vi "Main.vi"(11 "Module Admin":refnum<class "Delacor_lib_QMH_Module Admin.lvclass">) -> ()   [LabVIEW 2021, in "Sequence Engine.lvlib"]
doc: "This template is based off of the Queued Message Handler design pattern and the Queued Message Handler project template that ships with LabVIEW.\n\nThe main difference is that the queue is private to this module and communication between modules is performed via Broadcast and Request events.\n\nRequest events are wrapped in public API methods and are handled in the Event Handling Loop (EHL) of this VI. Any module can register for Broadcast events sent by this module. The EHL generates messages based on user interface actions.\n\nThe Message Handling Loop (MHL) processes messages generated by the EHL, or by other messages. The messages are string values, so new messages can be added easily to the Message Cases case structure in the MHL. Each message cluster can also provide an optional value for Message Data, which is a variant that can be converted to whatever message-specific data is required.\n_____\nBased on DQMH Dev Tools: Project Template 7.1.1.1528."
uses:
  Sequence Engine.lvlib
  <vilib>/Delacor/Delacor QMH/Libraries/Module Admin_class/Delacor_lib_QMH_Module Admin.lvclass
  Module Data--cluster.ctl
  Classes/Test Step/Test Step.lvclass
  Classes/Test Result/Test Result.lvclass
  Classes/Sequence Engine/Sequence Engine.lvclass
  Classes/Results Manager/Results Manager.lvclass
  Classes/UUT/UUT.lvclass
  <vilib>/Delacor/Delacor QMH/Libraries/Message Queue_class/Delacor_lib_QMH_Message Queue.lvclass/Delacor_lib_QMH_Message Queue.ctl
  Stop Argument--cluster.ctl
  <vilib>/Delacor/Delacor QMH/Libraries/Module Admin_class/Delacor_lib_QMH_Module Admin.lvclass/Delacor_lib_QMH_Module Admin.ctl
  REQ Run Sequence Argument--cluster.ctl
  Init Test Context Argument--cluster.ctl
  Sequence Context.ctl
  <vilib>/Utility/miscctls.llb/LVPointTypeDef.ctl
  Classes/Sequence Engine/Sequence Engine.lvclass/Sequence Engine.ctl
  Classes/UUT/UUT.lvclass/UUT.ctl
  Classes/Test Result/Result Data.ctl
  Classes/Test Result/Test Status.ctl
  Classes/Test Result/Test Result.lvclass/Test Result.ctl
  <vilib>/Delacor/Delacor QMH/Libraries/Message Queue_class/Delacor_lib_QMH_Enqueue Message (Single).vi
  <vilib>/Delacor/Delacor QMH/Libraries/Module Admin_class/Delacor_lib_QMH_Get External Launch.vi
  <vilib>/Delacor/Delacor QMH/Libraries/Message Queue_class/Delacor_lib_QMH_Message Queue.lvclass
  PPLs/Recipe.lvlibp/Classes/Recipe/Recipe.lvclass
panel:
  out "error out":errorcluster
  out "Status":string
  in  "Simulate MHL Error":bool
  in  "Simulate EHL Error":bool
  # "Other processes communicate with this Module via its Public API (wrappers for its Request Events).\n\nThis Module communicates with other processes via its Broadcast Events.\nAny process that wants to receive these messages can register for this module's Broadcast events."
  # "This template is for the DQMH framework. See the block diagram for more information on how to use this template."
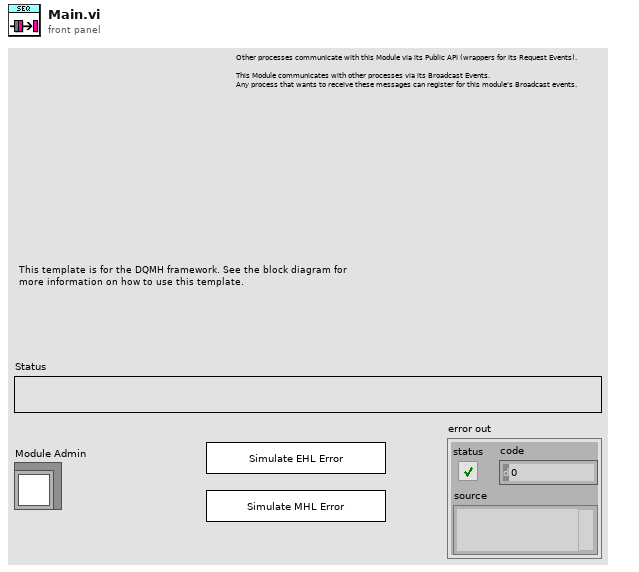
[diagram p1: front panel]
types:
  T1 = typedef "Sequence Engine.lvlib/Request Events--cluster.ctl" = cluster{"Stop Module":refnum<user-event>, "Show Panel":refnum<user-event>, "Hide Panel":refnum<user-event>, "Get Module Execution Status":refnum<user-event>, "Show Diagram":refnum<user-event>, "REQ Run Sequence":refnum<user-event>, "Request to stop testing":refnum<user-event>, "Init Test Context":refnum<user-event>}
  T2 = typedef "Sequence Engine.lvlib/Module Data--cluster.ctl" = cluster{"Steps Array":refnum<class "Test Step.lvclass">[], "Status":string, "Current Index":i32, "Current Step":refnum<class "Test Step.lvclass">, "Retried Count":u8, "Test Result":refnum<class "Test Result.lvclass">, "Sequence Engine":refnum<class "Sequence Engine.lvclass">, "Is Fail":bool, "Results Manager":refnum<class "Results Manager.lvclass">, "UUT.lvclass":refnum<class "UUT.lvclass">, "Run.Start JSON":string, "Test Aborted":bool}
  T3 = enum32{"invalid lock state", "Not Locked", "Locked (No Password)", "Password-protected"}
  T4 = typedef "Sequence Engine.lvlib/Stop Argument--cluster.ctl" = cluster{"Origin":string, "Exit via Stop Module Req?":bool, "Wait for Module to stop?":bool}
  T5 = typedef "Sequence Engine.lvlib/REQ Run Sequence Argument--cluster.ctl" = cluster{"Run.Start JSON":string}
  T6 = typedef "Sequence Engine.lvlib/Init Test Context Argument--cluster.ctl" = cluster{"Sequence Context":T7}
  T7 = typedef "Sequence Engine.lvlib/Sequence Engine.lvclass/Sequence Context.ctl" = cluster{"Execution Mode":enum16{"Production", "MSA1", "Trial"}, "Username":string, "Is Simulation":bool, "Hardware Map":string}
  T8 = typedef "LVPointTypeDef.ctl" = cluster{"Horizontal":i16, "Vertical":i16}
  T9 = enum32{"Invalid", "Standard", "Closed", "Hidden", "Minimized", "Maximized"}
  T10 = typedef "Sequence Engine.lvlib/Test Result.lvclass/Result Data.ctl" = cluster{"Test ID":u32, "Test Name":string, "Sub Test Name":string, "Test Status":T11, "Start Time":timestamp, "End Time":timestamp, "Duration (s)":dbl, "Expected Values":string, "Measured Values":string, "Remarks":string}
  T11 = typedef "Sequence Engine.lvlib/Test Result.lvclass/Test Status.ctl" = enum16{"Pass", "Fail", "Aborted", "Skipped"}
  T12 = typedef "Sequence Engine.lvlib/Test Factory.lvclass/Test Config.ctl" = cluster{"Test ID":string, "Test Name":string, "Test Group":string, "Enabled?":bool, "Timeout (s)":u16, "Retry Count":u16, "Recipe Parameters":string, "Sequence Config":string}
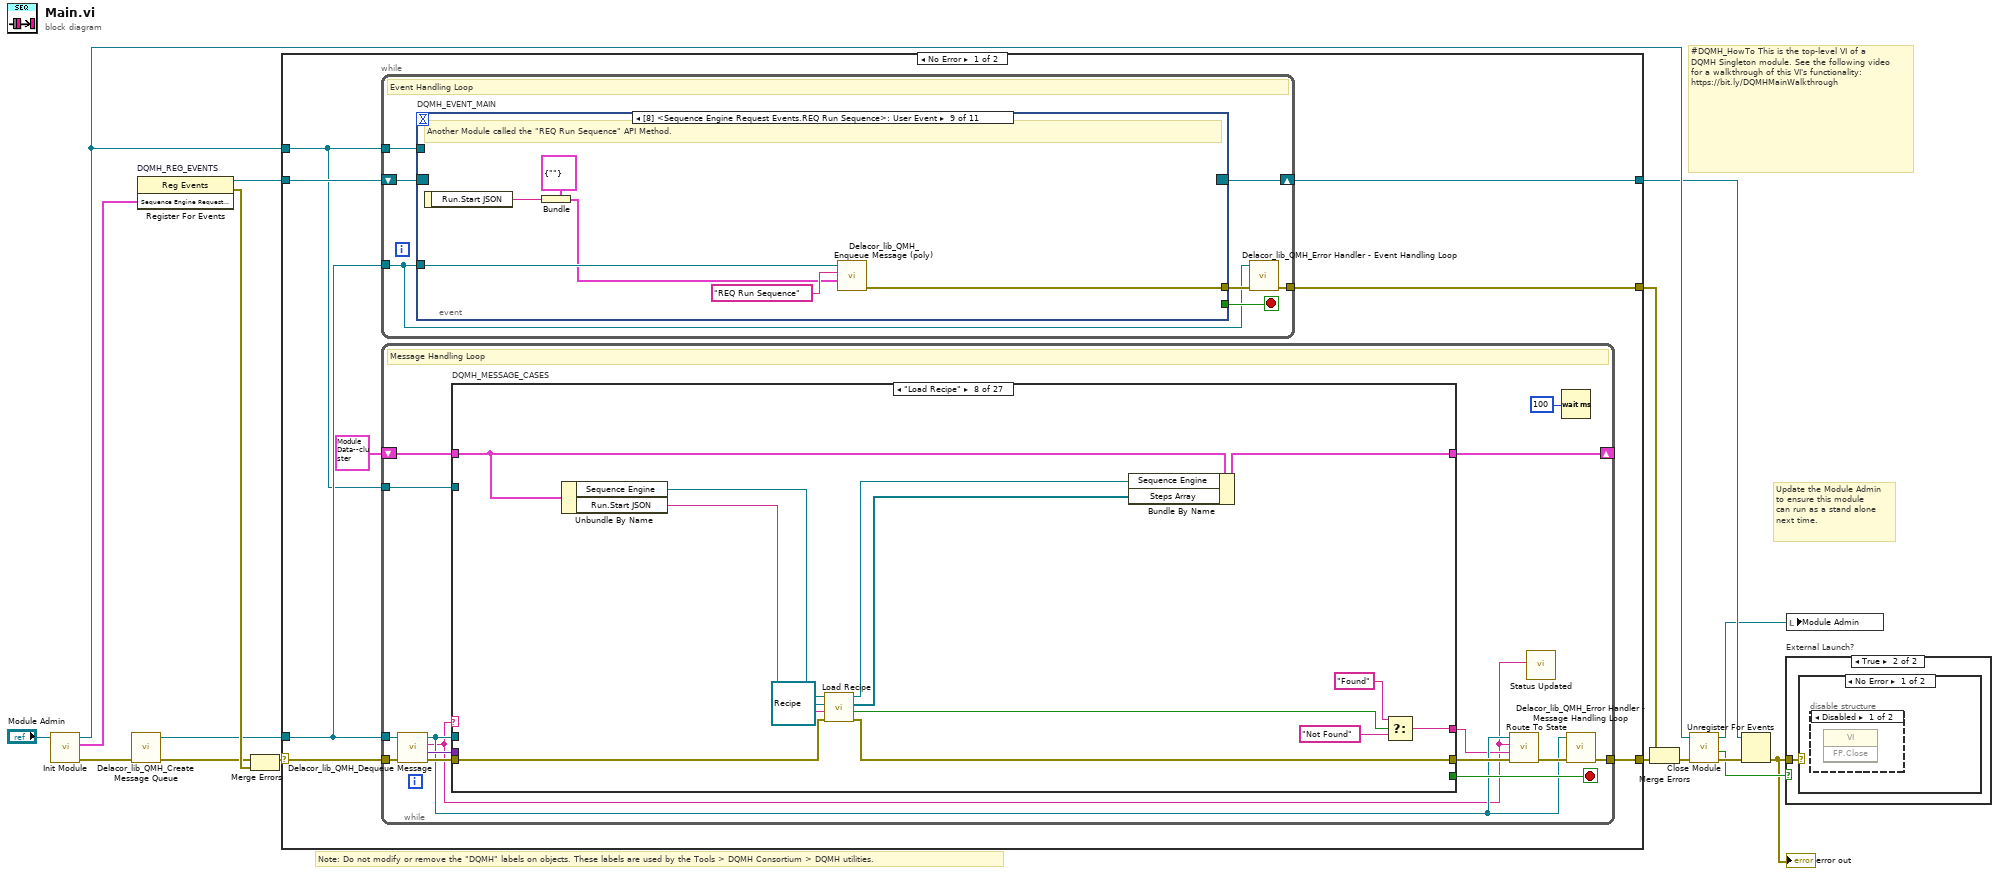
[diagram p0: block diagram]
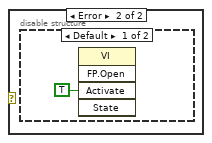
[diagram p4: hidden frame]
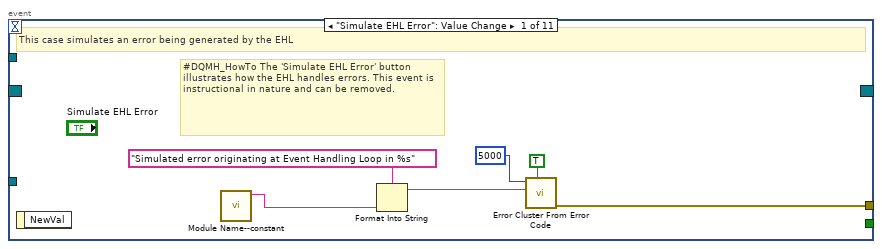
[diagram p6: hidden frame]
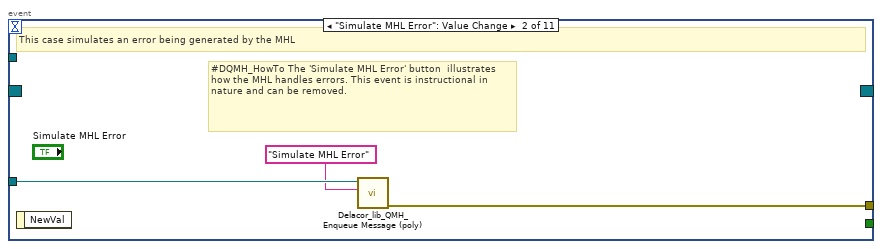
[diagram p7: hidden frame]
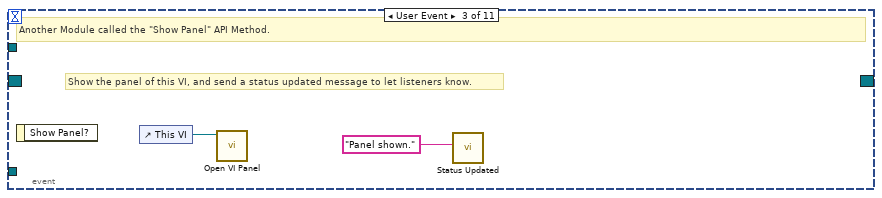
[diagram p8: hidden frame]
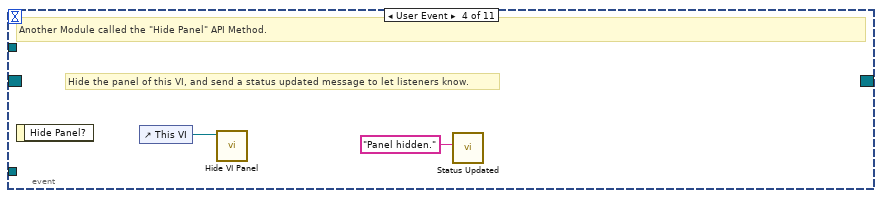
[diagram p9: hidden frame]
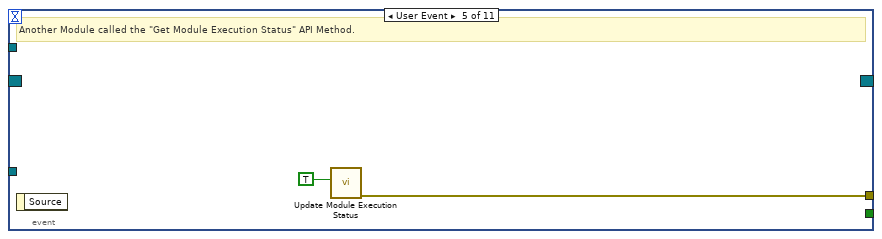
[diagram p10: hidden frame]
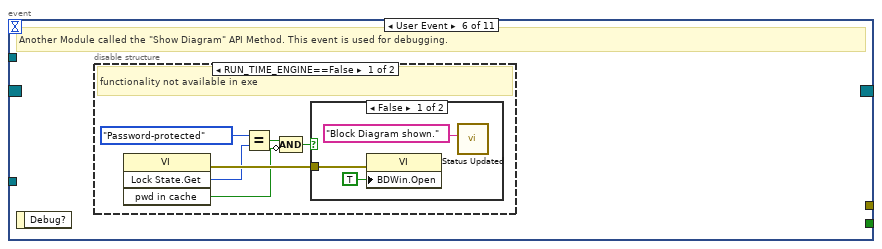
[diagram p11: hidden frame]
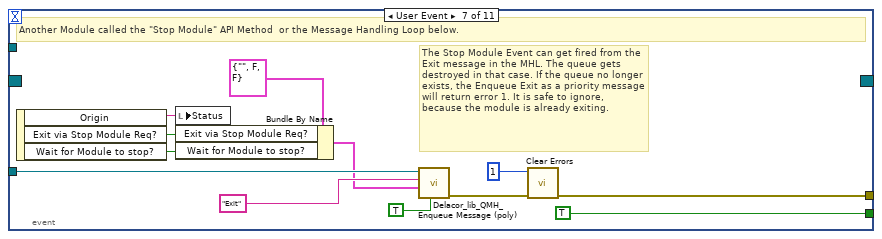
[diagram p14: hidden frame]
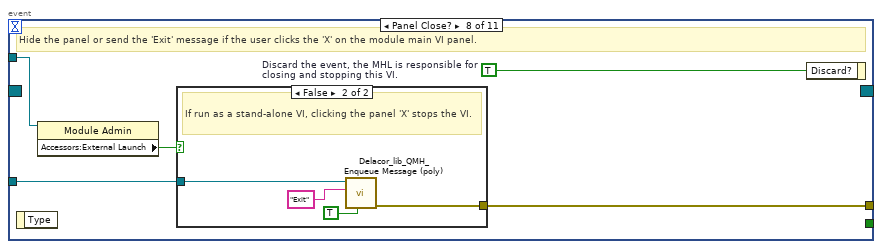
[diagram p15: hidden frame]
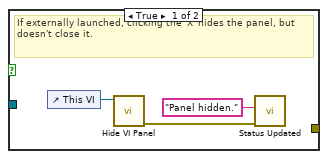
[diagram p16: hidden frame]
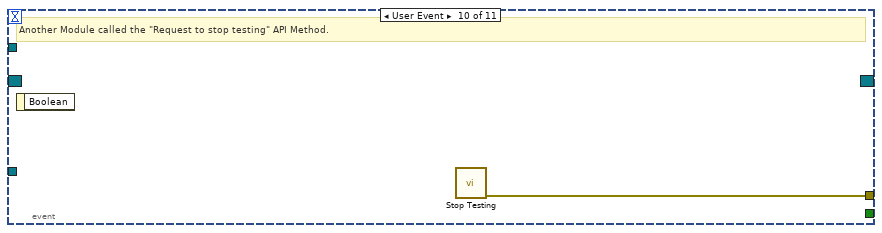
[diagram p17: hidden frame]
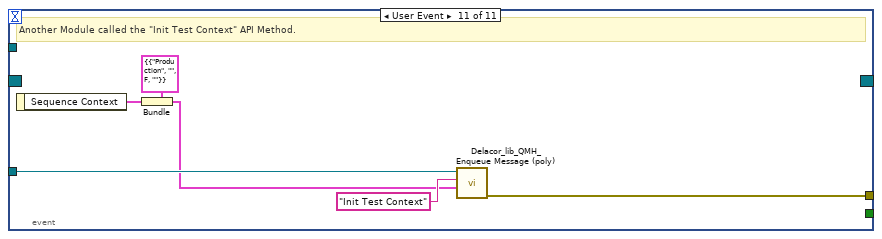
[diagram p18: hidden frame]
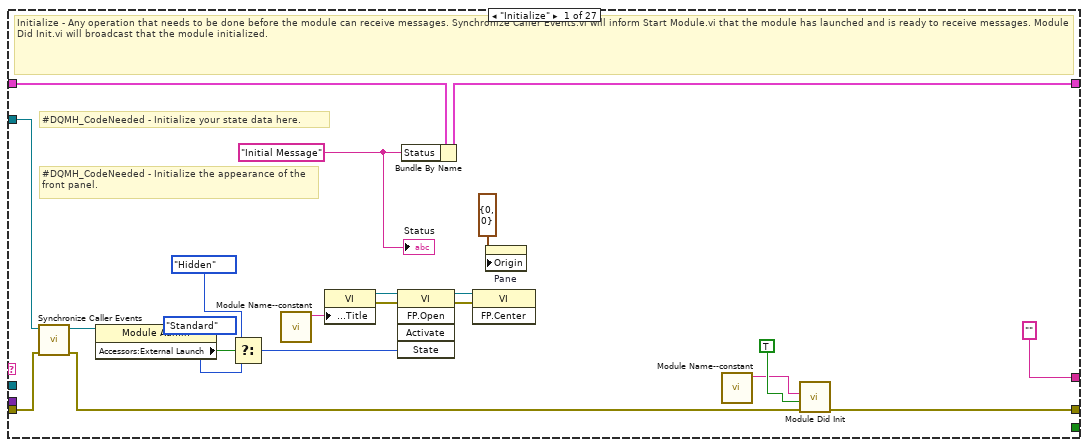
[diagram p19: hidden frame]
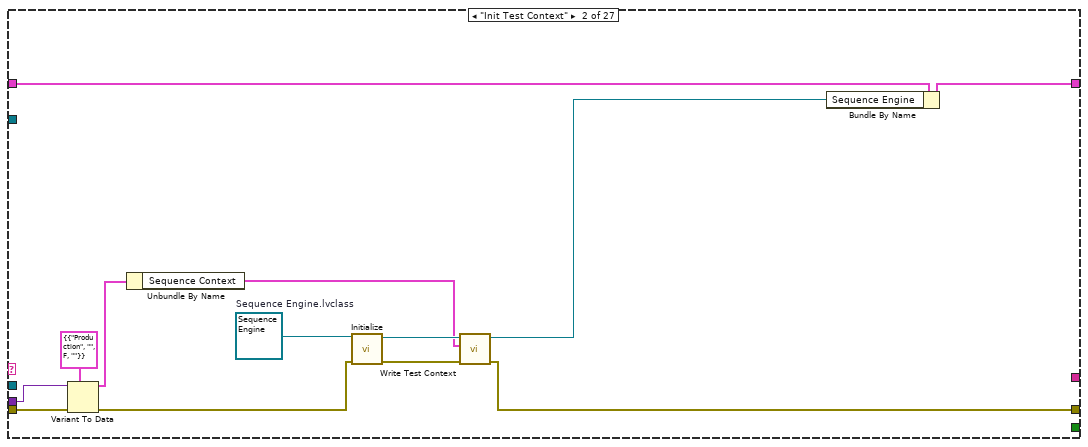
[diagram p20: hidden frame]
diagram:
  # "#DQMH_HowTo This is the top-level VI of a DQMH Singleton module. See the following video for a walkthrough of this VI's functionality: https://bit.ly/DQMHMainWalkthrough"
  # "Note: Do not modify or remove the \"DQMH\" labels on objects. These labels are used by the Tools > DQMH Consortium > DQMH utilities."
  # "Update the Module Admin to ensure this module can run as a stand alone next time."
  n1 = call "Init Module.vi"("Singleton Module Admin in"="Module Admin") -> ("error out"=w3:errorcluster, "Sequence Engine Request Events"=w8:T1, "Singleton Module Admin out"=w11:refnum<class "Delacor_lib_QMH_Module Admin.lvclass">)  [unwired: 8 in]
  n2 = call <vilib>:"Delacor_lib_QMH_Create Message Queue.vi"("error in"=w3) -> ("error out"=w2:errorcluster, "Message Queue"=w4:refnum<class "Delacor_lib_QMH_Message Queue.lvclass">)  [unwired: 9 in]
  n3 = register-events "DQMH_REG_EVENTS"(w8) -> (reference out=w9:refnum<event-registration>, error out=w12:errorcluster)  [unwired: 2 in]
  n4 = Merge Errors(w2, w12) -> (w13:errorcluster)
  n5 = case shown="No Error" w13 {
    selector: w13 -> [w23 w374]
    tunnel: [w25 w373] -> w17
    tunnel: [w22 w372] -> w10
    tunnel: w9 -> [w21 w372]
    tunnel: w4 -> [w20 w367]
    tunnel: [w24 _] -> w15
    tunnel: w11 -> [w19 w368]
    frame No Error {
      n6 = while {
        tunnel: w20 -> [w26]
        shift-right: [w29] -> w22
        shift-left: w21 -> [w30]
        tunnel: [w31] -> w24
        tunnel: w19 -> [w27]
        stop <- w28 stop-if-true
        # "Event Handling Loop"
        n7 = event "DQMH_EVENT_MAIN" shown="[8] <Sequence Engine Request Events.REQ Run Sequence>: User Event" {
          selector: w30 -> [_ _ _ _ _ _ _ _ _ _ _]
          dyn-events: [_ _ _ _ _ _ _ _ _ _ _] -> w29
          timeout: _ -> [_ _ _ _ _ _ _ _ _ _ _]
          tunnel: [_ _ _ _ _ _ TRUE ("Discard?") _ _ _ _] -> w28
          tunnel: w26 -> [_ w40 _ _ _ _ w64 w71 w86 _ w93]
          tunnel: [w38 w41 _ _ w47 _ w67 w73 w81 w87 w88] -> w32
          tunnel: w27 -> [_ _ _ _ _ _ _ w70 _ _ _]
          event "Simulate EHL Error": Value Change {
            # "#DQMH_HowTo The 'Simulate EHL Error' button  illustrates how the EHL handles errors. This event is instructional in nature and can be removed."
            # "This case simulates an error being generated by the EHL"
            n8 = event-data() -> ()  [unwired: 1 in, 1 out]
            n9 = call "Module Name--constant.vi"() -> ("Module Name"=w35:string)  [unwired: 11 in]
            n10 = Format Into String(format string="Simulated error originating at Event Handling Loop in %s", w35) -> (resulting string=w36:string)  [unwired: 2 in, 1 out]
            n11 = call <vilib>:"Error Cluster From Error Code.vi"("show call chain? (False)"=TRUE, "error message (\"\")"=w36, "error code (0)"=5000) -> ("error out"=w38:errorcluster)  [unwired: 6 in]
          }
          event "Simulate MHL Error": Value Change {
            # "#DQMH_HowTo The 'Simulate MHL Error' button  illustrates how the MHL handles errors. This event is instructional in nature and can be removed."
            # "This case simulates an error being generated by the MHL"
            n12 = event-data() -> ()  [unwired: 1 in, 1 out]
            n13 = call-poly <vilib>:"Delacor_lib_QMH_Enqueue Message (poly).vi"("Message"="Simulate MHL Error", "Message Queue in"=w40) -> ("error out"=w41:errorcluster)  [unwired: 8 in, 1 out]
          }
          event User Event {
            # "Show the panel of this VI, and send a status updated message to let listeners know."
            # "Another Module called the \"Show Panel\" API Method."
            n14 = event-data() -> ()  [unwired: 1 in, 1 out]
            n15 = control-ref of="This VI"() -> (w43:refnum<vi>)
            n16 = call "Open VI Panel.vi"("VI"=w43) -> ()  [unwired: 10 in, 1 out]
            n17 = call "Status Updated.vi"("Status"="Panel shown." ("format string")) -> ()  [unwired: 10 in, 1 out]
          }
          event User Event {
            # "Hide the panel of this VI, and send a status updated message to let listeners know."
            # "Another Module called the \"Hide Panel\" API Method."
            n18 = event-data() -> ()  [unwired: 1 in, 1 out]
            n19 = control-ref of="This VI"() -> (w45:refnum<vi>)
            n20 = call "Hide VI Panel.vi"("VI"=w45) -> ()  [unwired: 10 in, 1 out]
            n21 = call "Status Updated.vi"("Status"="Panel hidden." ("format string")) -> ()  [unwired: 10 in, 1 out]
          }
          event User Event {
            # "Another Module called the \"Get Module Execution Status\" API Method."
            n22 = event-data() -> ()  [unwired: 1 in, 1 out]
            n23 = call "Update Module Execution Status.vi"("Running?"=TRUE) -> ("error out"=w47:errorcluster)  [unwired: 10 in]
          }
          event User Event {
            # "Another Module called the \"Show Diagram\" API Method. This event is used for debugging."
            n24 = event-data() -> ()  [unwired: 1 in, 1 out]
            n25 = disable-structure shown="RUN_TIME_ENGINE==False" {
              frame condition #0 (active) {
                # "functionality not available in exe"
                n26 = invoke on="Invoke Node" class="VI" method="Lock State.Get"() -> (error out=w53:errorcluster, "Get Lock State"=w52:T3, "pwd in cache"=w49:bool)  [unwired: 4 in, 1 out]
                n27 = Equal?(x=T3."Password-protected", y=w52) -> (x = y?=w50:bool)
                n28 = Compound Arithmetic op=AND(w50, invert w49) -> (w48:bool)
                n29 = case shown="False" w48 {
                  tunnel: w53 -> [w56 _]
                  frame False {
                    n30 = property on="Property Node" class="VI"(error in=w56, "BDWin.Open"=TRUE ("Block Diagram Window:Open")) -> ()  [unwired: 1 in, 2 out]
                    n31 = call "Status Updated.vi"("Status"="Block Diagram shown." ("format string")) -> ()  [unwired: 10 in, 1 out]
                  }
                  frame True {
                    # "Password-protected VI, and the password is not in the cache. Do not show the diagram."
                  }
                }
              }
              frame condition #1 {
              }
            }
          }
          event User Event {
            # "The Stop Module Event can get fired from the Exit message in the MHL. The queue gets destroyed in that case. If the queue no longer exists, the Enqueue Exit as a priority message will return error 1. It is safe to ignore, because the module is already exiting."
            # "Another Module called the \"Stop Module\" API Method  or the Message Handling Loop below."
            n32 = event-data() -> ("Origin"=w63:string, "Exit via Stop Module Req?"=w59:bool, "Wait for Module to stop?"=w58:bool)  [unwired: 1 in]
            n33 = local write "Status"(w63) -> ()
            n34 = Bundle By Name(cluster=T4 {"Origin"="", "Exit via Stop Module Req?"=FALSE, "Wait for Module to stop?"=FALSE} ("Stop Argument"), "Exit via Stop Module Req?"=w59, "Wait for Module to stop?"=w58) -> (w57:T4)
            n35 = call-poly <vilib>:"Delacor_lib_QMH_Enqueue Message (poly).vi"("Priority Message? (F)"=TRUE, "Message Data"=w57, "Message"="Exit", "Message Queue in"=w64) -> ("error out"=w68:errorcluster)  [unwired: 6 in, 1 out]
            n36 = call <vilib>:"Clear Errors.vi"("error in (no error)"=w68, "specific error code to clear (0: all)"=1) -> ("error out"=w67:errorcluster)  [unwired: 4 in, 1 out]
          }
          event Panel Close? {
            w72 = TRUE  # Discard the event, the MHL is responsible for closing and stopping this VI.
            # "Hide the panel or send the 'Exit' message if the user clicks the 'X' on the module main VI panel."
            n37 = event-data() -> ()  [unwired: 1 in, 1 out]
            n38 = property on="Property Node" class="Module Admin"(reference=w70) -> ("Accessors:External Launch"=w69:bool)  [unwired: 1 in, 2 out]
            n39 = case shown="False" w69 {
              tunnel: w71 -> [_ w79]
              tunnel: [_ w80] -> w73
              frame True {
                # "If externally launched, clicking the 'X' hides the panel, but doesn't close it."
                n40 = control-ref of="This VI"() -> (w76:refnum<vi>)
                n41 = call "Hide VI Panel.vi"("VI"=w76) -> ("error out"=w74:errorcluster)  [unwired: 10 in]
                n42 = call "Status Updated.vi"("error in"=w74, "Status"="Panel hidden." ("format string")) -> ()  [unwired: 9 in, 1 out]
              }
              frame False {
                # "If run as a stand-alone VI, clicking the panel 'X' stops the VI."
                n43 = call-poly <vilib>:"Delacor_lib_QMH_Enqueue Message (poly).vi"("Priority Message? (F)"=TRUE, "Message"="Exit", "Message Queue in"=w79) -> ("error out"=w80:errorcluster)  [unwired: 7 in, 1 out]
              }
            }
            n44 = event-data ("Event Filter Node")("Discard?"=w72) -> ()  [unwired: 1 in, 1 out]
          }
          event User Event {
            # "Another Module called the \"REQ Run Sequence\" API Method."
            n45 = event-data() -> ("Run.Start JSON"=w82:string)  [unwired: 1 in]
            n46 = Bundle(cluster=T5 {"Run.Start JSON"=""} ("REQ Run Sequence Argument"), "Run.Start JSON"=w82) -> (w83:T5)
            n47 = call-poly <vilib>:"Delacor_lib_QMH_Enqueue Message (poly).vi"("Message Data"=w83, "Message"="REQ Run Sequence", "Message Queue in"=w86) -> ("error out"=w81:errorcluster)  [unwired: 7 in, 1 out]
          }
          event User Event {
            # "Another Module called the \"Request to stop testing\" API Method."
            n48 = event-data() -> ()  [unwired: 1 in, 1 out]
            n49 = call "Stop Testing.vi"() -> ("error out"=w87:errorcluster)  [unwired: 11 in]
          }
          event User Event {
            # "Another Module called the \"Init Test Context\" API Method."
            n50 = event-data() -> ("Sequence Context"=w89:T7)  [unwired: 1 in]
            n51 = Bundle(cluster=T6 {"Sequence Context"={"Execution Mode"=enum."Production", "Username"="", "Is Simulation"=FALSE, "Hardware Map"=""}} ("Init Test Context Argument"), "Sequence Context"=w89) -> (w90:T6)
            n52 = call-poly <vilib>:"Delacor_lib_QMH_Enqueue Message (poly).vi"("Message Data"=w90, "Message"="Init Test Context", "Message Queue in"=w93) -> ("error out"=w88:errorcluster)  [unwired: 7 in, 1 out]
          }
        }
        n53 = call-dynamic "Delacor_lib_QMH_Error Handler - Event Handling Loop.vi"("error in"=w32, "Message Queue in"=w26) -> ("dup error in"=w31:errorcluster)  [unwired: 8 in, 1 out]
      }
      n54 = while {
        tunnel: w20 -> [w100]
        shift-right: [w105] -> _
        shift-left: T2 {"Steps Array"=[], "Status"="", "Current Index"=0, "Current Step"=refnum, "Retried Count"=0, "Test Result"=refnum, "Sequence Engine"=refnum, "Is Fail"=FALSE, "Results Manager"=refnum, "UUT.lvclass"=refnum, "Run.Start JSON"="", "Test Aborted"=FALSE} ("Module Data") -> [w106]
        tunnel: w23 -> [w108]
        tunnel: [w101] -> w25
        tunnel: w19 -> [w102]
        stop <- w104 stop-if-true
        # "Message Handling Loop"
        n55 = call-dynamic "Delacor_lib_QMH_Dequeue Message.vi"("error in"=w108, "Message Queue in"=w100) -> ("error out"=w107:errorcluster, "Message Data"=w103:variant, "Message"=w95:string, "Message Queue out"=w97:refnum<class "Delacor_lib_QMH_Message Queue.lvclass">)  [unwired: 6 in]
        n56 = case "DQMH_MESSAGE_CASES" shown="\"Load Recipe\"" w95 {
          selector: w95 -> [_ _ _ _ _ _ _ _ _ _ _ _ _ _ _ _ _ _ _ _ _ _ _ _ _ _ w362]
          tunnel: w97 -> [_ _ _ _ _ _ _ _ _ _ _ _ _ _ _ _ _ _ _ _ _ _ _ _ w327 w351 _]
          tunnel: w107 -> [w127 w142 w144 w153 w157 w159 w162 w172 w182 w191 w203 w213 w227 w230 w248 w267 w275 w279 w295 w303 w309 w312 w314 w323 w334 w356 w365]
          tunnel: [w126 w130 w144 w152 w157 w159 w162 w171 w177 w191 w203 w213 w226 w229 w246 w262 w275 w278 w288 w302 w309 w311 w314 w322 w330 w341 w366] -> w99
          tunnel: w106 -> [w117 w141 w143 w155 w156 w158 w163 w176 w184 w190 w202 w212 w225 w242 w251 w272 w274 w282 w294 w307 w308 w310 w313 w320 w329 w342 w363]
          tunnel: [w116 w134 w143 w151 w156 w158 w161 w174 w181 w190 w201 w210 w223 w236 w247 w273 w274 w282 w289 w306 w308 w310 w313 w320 w329 w342 w363] -> w105
          tunnel: [_ _ _ _ _ _ _ _ _ _ _ _ _ _ _ _ _ _ _ _ _ _ _ _ _ w350 _] -> w104
          tunnel: w103 -> [_ w140 _ w147 _ _ _ _ _ _ _ _ _ _ _ _ _ _ _ _ _ _ _ _ w328 w349 _]
          tunnel: w102 -> [w118 _ _ _ _ _ _ _ _ _ _ _ _ _ _ _ _ _ _ _ _ _ _ _ w326 w344 _]
          tunnel: ["" ("Outcome") _ _ _ _ _ _ w168 _ _ w193 _ w218 w237 _ w255 _ w281 _ _ _ _ _ _ _ _ _] -> w96
          frame "Initialize" {
            w112 = "Initial Message" ("Initial Message")
            # "#DQMH_CodeNeeded - Initialize the appearance of the front panel."
            # "#DQMH_CodeNeeded - Initialize your state data here."
            # "Initialize - Any operation that needs to be done before the module can receive messages. Synchronize Caller Events.vi will inform Start Module.vi that the module has launched and is ready to receive messages. Module Did Init.vi will broadcast that the module initialized."
            n57 = call "Synchronize Caller Events.vi"("error in"=w127, "Singleton Module Admin in"=w118) -> ("error out"=w110:errorcluster, "Singleton Module Admin out"=w113:refnum<class "Delacor_lib_QMH_Module Admin.lvclass">)  [unwired: 8 in]
            n58 = property on="Property Node" class="Module Admin"(reference=w113) -> ("Accessors:External Launch"=w122:bool)  [unwired: 1 in, 2 out]
            n59 = Select(t=T9."Hidden" ("State"), s=w122, f=T9."Standard" ("State")) -> (s? t:f=w119:T9)
            n60 = call "Module Name--constant.vi"() -> ("Module Name"=w125:string)  [unwired: 11 in]
            n61 = property on="Property Node" class="VI"("Front Panel.Title"=w125) -> (reference out=w124:refnum<vi>, error out=w129:errorcluster)  [unwired: 2 in]
            n62 = invoke on="Invoke Node" class="VI" method="FP.Open"(reference=w124, error in=w129, "State"=w119) -> (reference out=w123:refnum<vi>, error out=w128:errorcluster)  [unwired: 2 in, 3 out]
            n63 = Bundle By Name(cluster=w117, "Status"=w112) -> (w116:T2)
            n64 = invoke on="Invoke Node" class="VI" method="FP.Center"(reference=w123, error in=w128) -> ()  [unwired: 1 in, 3 out]
            n65 = property on="Pane" class="Pane"("Origin"=T8 {"Horizontal"=0, "Vertical"=0}) -> ()  [unwired: 2 in, 2 out]
            n66 = call "Module Name--constant.vi"() -> ("Module Name"=w114:string)  [unwired: 11 in]
            n67 = call "Module Did Init.vi"("error in"=w110, "Initialized?"=TRUE, "Origin"=w114) -> ("error out"=w126:errorcluster)  [unwired: 8 in]
            "Status" <- w112
          }
          frame "Init Test Context" {
            w135 = refnum<class "Sequence Engine.lvclass"> refnum  # Sequence Engine.lvclass
            n68 = Variant To Data(error in=w142, type=T6 {"Sequence Context"={"Execution Mode"=enum."Production", "Username"="", "Is Simulation"=FALSE, "Hardware Map"=""}} ("Init Test Context Argument"), Variant=w140) -> (data=w138:T6, error out=w132:errorcluster)
            n69 = Unbundle By Name(w138) -> ("Sequence Context"=w131:T7)
            n70 = call "Initialize.vi"("error in (no error)"=w132, "Sequence Engine in"=w135) -> ("error out"=w137:errorcluster, "Sequence Engine out"=w136:refnum<class "Sequence Engine.lvclass">)  [unwired: 8 in]
            n71 = call "Write Test Context.vi"("error in (no error)"=w137, "Test Context"=w131, "Sequence Engine in"=w136) -> ("error out"=w130:errorcluster, "Sequence Engine out"=w133:refnum<class "Sequence Engine.lvclass">)  [unwired: 7 in]
            n72 = Bundle By Name(cluster=w141, "Sequence Engine"=w133) -> (w134:T2)
          }
          frame "---Module Specific---" {
            # "Separator -- The following cases handle messages specific to this Module."
          }
          frame "REQ Run Sequence" {
            n73 = Variant To Data(error in=w153, type=T5 {"Run.Start JSON"=""} ("REQ Run Sequence Argument"), Variant=w147) -> (data=w146:T5, error out=w149:errorcluster)
            n74 = Unbundle By Name(w146) -> ("Run.Start JSON"=w145:string)
            n75 = Unbundle By Name(w155) -> ("Sequence Engine"=w154:refnum<class "Sequence Engine.lvclass">)
            n76 = call "Run.vi"("error in (no error)"=w149, "Sequence Engine in"=w154) -> ("error out"=w152:errorcluster, "Sequence Engine out"=w150:refnum<class "Sequence Engine.lvclass">)  [unwired: 8 in]
            n77 = Bundle By Name(cluster=w155, "Sequence Engine"=w150, "Run.Start JSON"=w145) -> (w151:T2)
          }
          frame "---Sequence Specific---" {
            # "Separator -- The following cases handle messages specific to this Test Sequence"
          }
          frame "--- UUT Loop starts ----" {
          }
          frame "Pre Sequence Run" {
            n78 = Bundle By Name(cluster=w163, "Current Index"=0) -> (w161:T2)
          }
          frame "Load Recipe" {
            n79 = Unbundle By Name(w176) -> ("Sequence Engine"=w175:refnum<class "Sequence Engine.lvclass">, "Run.Start JSON"=w169:string)
            n80 = call "Load Recipe.vi"("error in (no error)"=w172, "Run.Start JSON"=w169, "Recipe.lvclass"=refnum<class "Recipe.lvclass"> refnum, "Sequence Engine in"=w175) -> ("error out"=w171:errorcluster, "Found?"=w165:bool, "Steps Array"=w173:refnum<class "Test Step.lvclass">[], "Sequence Engine out"=w170:refnum<class "Sequence Engine.lvclass">)  [unwired: 4 in]
            n81 = Bundle By Name(cluster=w176, "Sequence Engine"=w170, "Steps Array"=w173) -> (w174:T2)
            n82 = Select(t="Found", s=w165, f="Not Found") -> (s? t:f=w168:string)
          }
          frame "Insert Report Header" {
            n83 = Unbundle By Name(w184) -> ("Sequence Engine"=w183:refnum<class "Sequence Engine.lvclass">, "UUT.lvclass"=w179:refnum<class "UUT.lvclass">)
            n84 = disable-structure shown="Disabled" {
              disable-tunnel: w183 -> [w189 _]
              disable-tunnel: w182 -> [w188 _]
              disable-tunnel: [w187 _] -> w180
              disable-tunnel: w179 -> [w186 _]
              disable-tunnel: [w185 _] -> w178
              frame Disabled {
                n85 = call "Create Report Header.vi"("error in (no error)"=w188, "UUT.lvclass"=w186, "Sequence Engine in"=w189) -> ("error out"=w185:errorcluster, "Sequence Engine out"=w187:refnum<class "Sequence Engine.lvclass">)  [unwired: 6 in, 1 out]
              }
              frame Enabled {
              }
            }
            n86 = call "Testing Started.vi"("error in"=w178) -> ("error out"=w177:errorcluster)  [unwired: 10 in]
            n87 = Bundle By Name(cluster=w184, "Sequence Engine"=w180) -> (w181:T2)
          }
          frame "--- Test Loop starts ----" {
          }
          frame "Sequence Iterator" {
            n88 = Unbundle By Name(w202) -> ("Steps Array"=w199:refnum<class "Test Step.lvclass">[], "Current Index"=w198:i32)
            n89 = Index Array(array=w199, index=w198) -> (element=w200:refnum<class "Test Step.lvclass">)
            n90 = Array Size(array=w199) -> (size(s)=w197:i32)
            n91 = Less?(x=w198, y=w197) -> (x < y?=w196:bool)
            n92 = Select(t="Pre Test", s=w196, f="Completed") -> (s? t:f=w193:string)
            n93 = Bundle By Name(cluster=w202, "Retried Count"=u8 0, "Current Step"=w200) -> (w201:T2)
          }
          frame "Pre Test Run" {
            n94 = Unbundle By Name(w212) -> ("Current Step"=w211:refnum<class "Test Step.lvclass">)
            n95 = Get Date/Time In Seconds() -> (seconds since 1Jan1904=w205:timestamp)
            n96 = Bundle By Name(cluster=T10 {"Test ID"=0, "Test Name"="", "Sub Test Name"="", "Test Status"=enum."Pass", "Start Time"=timestamp(0 s since 1904-01-01), "End Time"=timestamp(0 s since 1904-01-01), "Duration (s)"=0.0, "Expected Values"="", "Measured Values"="", "Remarks"=""} ("Result Data"), "Start Time"=w205) -> (w206:T10)
            n97 = call "Write Result Data.vi"("Result Data"=w206, "Test Result in"=refnum<class "Test Result.lvclass"> refnum ("Test Result.lvclass")) -> ("Test Result out"=w204:refnum<class "Test Result.lvclass">)  [unwired: 8 in, 1 out]
            n98 = call-dynamic "Init Test Result Data.vi"("Result.lvclass"=w204, "Test Step in"=w211) -> ("Test Step out"=w209:refnum<class "Test Step.lvclass">)  [unwired: 8 in, 1 out]
            n99 = Bundle By Name(cluster=w212, "Current Step"=w209) -> (w210:T2)
          }
          frame "Execute Test" {
            n100 = Unbundle By Name(w225) -> ("Current Step"=w224:refnum<class "Test Step.lvclass">)
            n101 = call-dynamic "Execute.vi"("error in (no error)"=w227, "Test Step in"=w224) -> ("error out"=w226:errorcluster, "Test Result"=w221:refnum<class "Test Result.lvclass">, "Test Step out"=w222:refnum<class "Test Step.lvclass">)  [unwired: 7 in]
            n102 = call "Read Result Data.vi"("Test Result in"=w221) -> ("Result Data"=w219:T10)  [unwired: 8 in, 2 out]
            n103 = Unbundle By Name(w219) -> ("Test Status"=w215:T11)
            n104 = call "New Test Result.vi"("Result Data"=w219) -> ()  [unwired: 10 in, 1 out]
            n105 = Equal?(x=Test_Status."Aborted", y=w215) -> (x = y?=w214:bool)
            n106 = Equal?(x=Test_Status."Fail", y=w215) -> (x = y?=w217:bool)
            n107 = Bundle By Name(cluster=w225, "Current Step"=w222, "Test Result"=w221, "Test Aborted"=w214, "Is Fail"=w217) -> (w223:T2)
            n108 = Format Into String(w215) -> (resulting string=w218:string)  [unwired: 3 in, 1 out]
          }
          frame "Test Fail" {
            n109 = Unbundle By Name(w242) -> ("Retried Count"=w233:u8, "Current Step"=w241:refnum<class "Test Step.lvclass">)
            n110 = call-dynamic "Read Step Config.vi"("error in (no error)"=w230, "Test Step in"=w241) -> ("Step Config"=w240:T12)  [unwired: 7 in, 2 out]
            n111 = Unbundle By Name(w240) -> ("Retry Count"=w228:u16)
            n112 = To Unsigned Word Integer(number=w233) -> (unsigned 16bit integer=w231:u16)
            n113 = call "Retried Count.vi"("error in"=w230, "Retried Count"=w228) -> ("error out"=w229:errorcluster)  [unwired: 9 in]
            n114 = Greater?(x=w228, y=w231) -> (0:w235:bool)
            n115 = Increment(x=w233) -> (x+1=w234:u8)
            n116 = Select(t="Retry", s=w235, f="Don't Retry") -> (s? t:f=w237:string)
            n117 = Select(t=w234, s=w235, f=w233) -> (s? t:f=w232:u8)
            n118 = Bundle By Name(cluster=w242, "Retried Count"=w232) -> (w236:T2)
          }
          frame "Save Test Result" {
            n119 = Unbundle By Name(w251) -> ("Sequence Engine"=w245:refnum<class "Sequence Engine.lvclass">, "Test Aborted"=w243:bool, "Current Step"=w250:refnum<class "Test Step.lvclass">)
            n120 = disable-structure shown="Disabled" {
              disable-tunnel: w250 -> [w254 _]
              disable-tunnel: [w253 _] -> w249
              disable-tunnel: w248 -> [w252 _]
              frame Disabled {
                n121 = call-dynamic "Save Test Result.vi"("error in (no error)"=w252, "Test Step in"=w254) -> ("error out"=w253:errorcluster)  [unwired: 8 in, 1 out]
              }
              frame Enabled {
              }
            }
            n122 = call "Write Is Aborted.vi"("error in (no error)"=w249, "Is Aborted"=w243, "Sequence Engine in"=w245) -> ("error out"=w246:errorcluster, "Sequence Engine out"=w244:refnum<class "Sequence Engine.lvclass">)  [unwired: 7 in]
            n123 = Bundle By Name(cluster=w251, "Sequence Engine"=w244) -> (w247:T2)
          }
          frame "Post Test Run" {
            n124 = Unbundle By Name(w272) -> ("Current Index"=w271:i32, "Results Manager"=w269:refnum<class "Results Manager.lvclass">, "Test Result"=w268:refnum<class "Test Result.lvclass">, "Sequence Engine"=w266:refnum<class "Sequence Engine.lvclass">, "Test Aborted"=w257:bool, "Is Fail"=w261:bool)
            n125 = Increment(x=w271) -> (x+1=w270:i32)
            n126 = call-dynamic "Add Result.vi"("error in (no error)"=w267, "Test Result.lvclass"=w268, "Results Manager in"=w269) -> ("error out"=w263:errorcluster, "Results Manager out"=w265:refnum<class "Results Manager.lvclass">)  [unwired: 7 in]
            n127 = call "Write Results Manager.vi"("error in (no error)"=w263, "Results Manager.lvclass"=w265, "Sequence Engine in"=w266) -> ("error out"=w262:errorcluster, "Sequence Engine out"=w264:refnum<class "Sequence Engine.lvclass">)  [unwired: 7 in]
            n128 = Bundle By Name(cluster=w272, "Current Index"=w270, "Results Manager"=w265, "Sequence Engine"=w264) -> (w273:T2)
            n129 = Select(t="Test Fail", s=w261, f="Not Fail") -> (s? t:f=w258:string)
            n130 = Select(t="Test Aborted", s=w257, f=w258) -> (s? t:f=w255:string)
          }
          frame "--- Test Loop stops ----" {
          }
          frame "Check Execution Mode" {
            n131 = Unbundle By Name(w282) -> ("Sequence Engine"=w280:refnum<class "Sequence Engine.lvclass">)
            n132 = call "Read Test Context.vi"("error in (no error)"=w279, "Sequence Engine in"=w280) -> ("error out"=w278:errorcluster, "Test Context"=w277:T7)  [unwired: 7 in, 1 out]
            n133 = Unbundle By Name(w277) -> ("Execution Mode"=w276:enum16{"Production", "MSA1", "Trial"})
            n134 = case shown="\"Production\", Default" w276 {
              tunnel: ["Production"] -> w281
              frame "Production", Default {
              }
            }
          }
          frame "Save Final Result" {
            n135 = Unbundle By Name(w294) -> ("Results Manager"=w290:refnum<class "Results Manager.lvclass">, "Sequence Engine"=w292:refnum<class "Sequence Engine.lvclass">, "UUT.lvclass"=w284:refnum<class "UUT.lvclass">)
            n136 = disable-structure shown="Disabled" {
              disable-tunnel: w295 -> [w300 _]
              disable-tunnel: [w299 _] -> w293
              disable-tunnel: w292 -> [w298 _]
              disable-tunnel: [w297 _] -> w287
              disable-tunnel: w284 -> [w296 _]
              frame Disabled {
                n137 = call "Log Report.vi"("error in (no error)"=w300, "UUT.lvclass"=w296, "Sequence Engine in"=w298) -> ("error out"=w299:errorcluster, "Sequence Engine out"=w297:refnum<class "Sequence Engine.lvclass">)  [unwired: 6 in, 1 out]
              }
              frame Enabled {
              }
            }
            n138 = call "Clear Results.vi"("error in (no error)"=w293, "Results Manager in"=w290) -> ("error out"=w291:errorcluster, "Results Manager out"=w285:refnum<class "Results Manager.lvclass">)  [unwired: 8 in]
            n139 = call "Write Results Manager.vi"("error in (no error)"=w291, "Results Manager.lvclass"=w285, "Sequence Engine in"=w287) -> ("error out"=w288:errorcluster, "Sequence Engine out"=w286:refnum<class "Sequence Engine.lvclass">)  [unwired: 7 in]
            n140 = Bundle By Name(cluster=w294, "Results Manager"=w285, "Sequence Engine"=w286) -> (w289:T2)
          }
          frame "Post Sequence Run" {
            n141 = Bundle By Name(cluster=w307, "Current Index"=0, "Is Fail"=FALSE, "Test Aborted"=FALSE) -> (w306:T2)
            n142 = call "Testing Completed.vi"("error in"=w303) -> ("error out"=w302:errorcluster)  [unwired: 10 in]
          }
          frame "--- UUT Loop stops ----" {
          }
          frame "---Copy This Frame---" {
            # "Duplicate this frame when creating new messages.  Change this comment in the duplicated frame to describe this message."
            n143 = Merge Errors(w312) -> (w311:errorcluster)
          }
          frame "---Exit and Error Handling---" {
            # "Separator - The following cases handle errors and exit messages."
          }
          frame "Simulate MHL Error" {
            # "#DQMH_HowTo The 'Simulate MHL Error' button  illustrates how the MHL handles errors. This event is instructional in nature and can be removed."
            # "Simulate an error occurring at the MHL"
            n144 = call "Module Name--constant.vi"() -> ("Module Name"=w316:string)  [unwired: 11 in]
            n145 = Format Into String(format string="Simulated error originating at Message Handling Loop in %s", w316) -> (resulting string=w317:string)  [unwired: 2 in, 1 out]
            n146 = call <vilib>:"Error Cluster From Error Code.vi"("show call chain? (False)"=TRUE, "error message (\"\")"=w317, "error code (0)"=5001) -> ("error out"=w321:errorcluster)  [unwired: 6 in]
            n147 = Merge Errors(w323, w321) -> (w322:errorcluster)
          }
          frame "Error" {
            # "#DQMH_CodeRecommended - If the module is running in standalone mode (External Launch = FALSE), this code will pop up an error dialog and call the 'Exit' message if an error occurs. Add more fine-grained error management here."
            # "Error - Check the error message data and respond accordingly. This message is sent by the \"Error Handler\" VIs at the end of each loop in this application."
            n148 = property on="Property Node" class="Module Admin"(reference=w326) -> ("Accessors:External Launch"=w325:bool)  [unwired: 1 in, 2 out]
            n149 = Variant To Data(error in=w334, type=errorcluster {"status"=FALSE, "code"=0, "source"=""} ("error constant"), Variant=w328) -> (data=w324:errorcluster, error out=w332:errorcluster)
            n150 = local write "error out"(w324) -> ()
            n151 = call "Error Reported.vi"("Error"=w324) -> ()  [unwired: 10 in, 1 out]
            n152 = case shown="True" w325 {
              tunnel: [w339 _] -> w331
              tunnel: w327 -> [w337 _]
              tunnel: w324 -> [w338 _]
              frame False {
                n153 = disable-structure shown="Default" {
                  disable-tunnel: w338 -> [w340 _]
                  frame condition #0 (active) {
                    # "If the module is running standalone, then pop up an error dialog and call the \"Exit\" message."
                    n154 = call <vilib>:"Simple Error Handler.vi"("error in (no error)"=w340) -> ()  [unwired: 4 in, 5 out]
                  }
                  frame condition #1 {
                    # "To prevent the Simple Error Handler VI from being loaded (e.g. when deploying to a Real-Time target), add the Conditional Disable Symbol \"DQMH_Disable_SEH\" to your project and set it to TRUE."
                  }
                }
                n155 = call-poly <vilib>:"Delacor_lib_QMH_Enqueue Message (poly).vi"("Priority Message? (F)"=TRUE, "Message"="Exit", "Message Queue in"=w337) -> ("error out"=w339:errorcluster)  [unwired: 7 in, 1 out]
              }
              frame True {
                n156 = call "Module Name--constant.vi"() -> ()  [unwired: 11 in, 1 out]
              }
            }
            n157 = Merge Errors(w332, w331) -> (w330:errorcluster)
          }
          frame "Exit" {
            w348 = 91  # 91: not all Exit messages will have an argument
            w350 = TRUE  # Stop the VI
            # "Release the message queue reference"
            # "Exit - Exit the application."
            n158 = Variant To Data(error in=w356, type=T4 {"Origin"="", "Exit via Stop Module Req?"=FALSE, "Wait for Module to stop?"=FALSE} ("Stop Argument"), Variant=w349) -> (data=w346:T4, error out=w353:errorcluster)
            n159 = call <vilib>:"Clear Errors.vi"("error in (no error)"=w353, "specific error code to clear (0: all)"=w348) -> ("error out"=w355:errorcluster)  [unwired: 4 in, 1 out]
            n160 = control-ref of="This VI"() -> (w345:refnum<vi>)
            n161 = call-dynamic "Delacor_lib_QMH_Release Message Queue.vi"("error in"=w355, "Message Queue"=w351) -> ("error out"=w354:errorcluster)  [unwired: 9 in]
            n162 = call "Handle Exit.vi"("Stop Argument"=w346, "Admin in"=w344, "VI reference"=w345) -> ("error out"=w352:errorcluster)  [unwired: 7 in, 1 out]
            n163 = Merge Errors(w354, w352) -> (w343:errorcluster)
            n164 = call "Error Reported.vi"("Error"=w343) -> ()  [unwired: 10 in, 1 out]
            n165 = Merge Errors(w343) -> (w341:errorcluster)
          }
          frame Default {
            # "'Default' case only runs if there is a message that isn't defined in any of the other cases.  Output a programming error."
            n166 = call "Module Name--constant.vi"() -> ("Module Name"=w361:string)  [unwired: 11 in]
            n167 = Format Into String(format string="The invalid message string \"%s\" was received in the Message Handling Loop for module \"%s\".", w362, w361) -> (resulting string=w357:string)  [unwired: 2 in, 1 out]
            n168 = call <vilib>:"Error Cluster From Error Code.vi"("show call chain? (False)"=TRUE, "error message (\"\")"=w357, "error code (0)"=1) -> ("error out"=w364:errorcluster)  [unwired: 6 in]
            n169 = Merge Errors(w365, w364) -> (w366:errorcluster)
          }
        }
        n170 = call "Route To State.vi"("error in"=w99, "Outcome"=w96, "Current State"=w95, "Message Queue in"=w97) -> ("error out"=w98:errorcluster)  [unwired: 7 in]
        n171 = call "Status Updated.vi"("Status"=w95) -> ()  [unwired: 10 in, 1 out]
        n172 = Wait (ms)(milliseconds to wait=u32 100) -> ()  [unwired: 1 out]
        n173 = call-dynamic "Delacor_lib_QMH_Error Handler - Message Handling Loop.vi"("error in"=w98, "Message Queue in"=w97) -> ("dup error in"=w101:errorcluster)  [unwired: 8 in, 1 out]
      }
    }
    frame Error {
      # "Synchronize Caller Events.vi will inform Start Module.vi that the module has launched and will let the code calling Start Module.vi register for broadcasts and would permit the caller receive the broadcast that an error occurred at launch time."
      n174 = call-dynamic "Delacor_lib_QMH_Release Message Queue.vi"("error in"=w374, "Message Queue"=w367) -> ("error out"=w373:errorcluster)  [unwired: 9 in]
      n175 = call "Synchronize Caller Events.vi"("Singleton Module Admin in"=w368) -> ("error out"=w375:errorcluster)  [unwired: 9 in, 1 out]
      n176 = call "Module Name--constant.vi"() -> ("Module Name"=w371:string)  [unwired: 11 in]
      n177 = Format Into String(format string="An error occurred during initialization. %s is no longer running.", w371) -> (resulting string=w369:string)  [unwired: 2 in, 1 out]
      n178 = Merge Errors(w373, w375) -> (w376:errorcluster)
      n179 = call "Error Reported.vi"("Additional Information"=w369, "Error"=w376) -> ()  [unwired: 9 in, 1 out]
    }
  }
  n180 = Merge Errors(w15, w17) -> (w14:errorcluster)
  n181 = call "Close Module.vi"("error in"=w14, "Module Admin in"=w11) -> ("error out"=w16:errorcluster, "External Launch"=w5:bool, "Module Admin out"=w6:refnum<class "Delacor_lib_QMH_Module Admin.lvclass">)  [unwired: 7 in]
  n182 = Unregister For Events(event registration refnum=w10, error in=w16) -> (error out=w1:errorcluster)
  "error out" <- w1
  n183 = case "External Launch?" shown="True" w5 {
    tunnel: w1 -> [_ w377]
    frame False {
    }
    frame True {
      n184 = case shown="No Error" w377 {
        frame No Error {
          n185 = disable-structure shown="Disabled" {
            frame Disabled {
              n186 = invoke on="Invoke Node" class="VI" method="FP.Close"() -> ()  [unwired: 3 in, 3 out]
            }
            frame Enabled {
            }
          }
        }
        frame Error {
          n187 = disable-structure shown="Default" {
            frame condition #0 (active) {
              n188 = invoke class="VI" method="FP.Open"("Activate"=TRUE ("Activate?")) -> ()  [unwired: 4 in, 5 out]
            }
            frame condition #1 {
              # "Don't show panel on error if running inside a built EXE."
            }
          }
        }
      }
    }
  }
  n189 = local write "Module Admin"(w6) -> ()
